vi "CheckIfInLimits.vi"(9 "Value":string, 10 "ID":u16, 11 "Parameter List":T2(array[cluster])) -> (1 "plValue":i32, 2 "Cluster":T1, 3 "Boolean":bool)   [LabVIEW 2023, in "ZWO_ASI.lvlib" / "ZWO_ASI.lvclass"]
uses:
  ZWO_ASI.lvclass
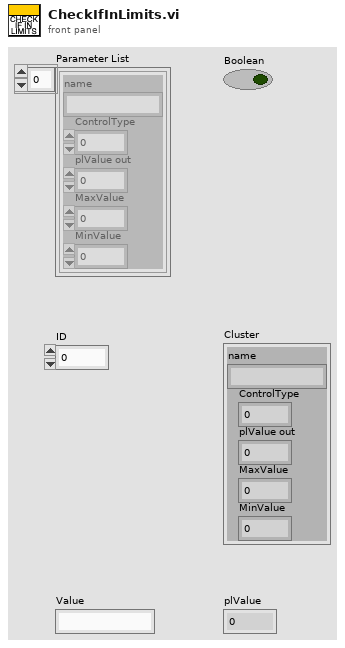
[diagram p1: front panel]
types:
  T1 = cluster{"name":string, "ControlType":u32, "plValue out":i32, "MaxValue":i32, "MinValue":i32}
  T2 = cluster{"name":string, "ControlType":u32, "plValue out":i32, "MaxValue":i32, "MinValue":i32}[]
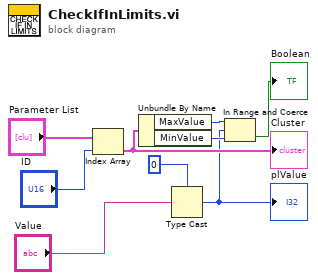
[diagram p0: block diagram]
diagram:
  n1 = Index Array(array="Parameter List", index="ID") -> (element=w4:T1)
  "Cluster" <- w4
  n2 = Unbundle By Name(w4) -> ("MaxValue"=w5:i32, "MinValue"=w6:i32)
  n3 = Type Cast(type=0 ("plValue"), x="Value") -> (*(type *) &x=w3:i32)
  "plValue" <- w3
  n4 = In Range and Coerce(upper limit=w5, x=w3, lower limit=w6) -> (In Range?=→"Boolean":bool)  [unwired: 1 out]
